vi "Create Initialization File.vi"   [LabVIEW 2015]
uses:
  Resources/Type Defs/Default Settings.ctl
  <vilib>/Utility/xml.llb/Write to XML File(string).vi
panel:
  # "Open the Block Diagram (Ctrl-E)\nto edit initialization settings."
types:
  T1 = typedef "Default Settings.ctl" = cluster{"Refresh Timeout (ms)":i32, "Version String":string, "Hardware Configuration File":string}
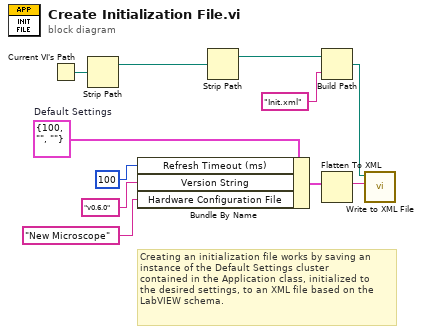
[diagram p0: block diagram]
diagram:
  w1 = T1 {"Refresh Timeout (ms)"=100, "Version String"="", "Hardware Configuration File"=""}  # Default Settings
  # "Creating an initialization file works by saving an\ninstance of the Default Settings cluster\ncontained in the Application class, initialized to \nthe desired settings, to an XML file based on the \nLabVIEW schema."
  n1 = Current VI's Path() -> (path=w7:path)
  n2 = Strip Path(path=w7) -> (stripped path=w6:path)  [unwired: 1 out]
  n3 = Bundle By Name(cluster=w1, "Refresh Timeout (ms)"=100, "Version String"="v0.6.0", "Hardware Configuration File"="New Microscope") -> (w11:T1)
  n4 = Strip Path(path=w6) -> (stripped path=w5:path)  [unwired: 1 out]
  n5 = Build Path(base path=w5, name or relative path="Init.xml") -> (appended path=w3:path)
  n6 = Flatten To XML(anything=w11) -> (xml string=w10:string)
  n7 = call-poly <vilib>:"Write to XML File.vi"("XML Input"=w10, "XML File Path"=w3) -> ()  [unwired: 7 in, 3 out]
